vi "Curtin1_Search.vi"(9 "Old Files":T3[](array[typedef])) -> (1 "New Files":T3[](array[typedef]), 3 "Ok?":bool)   [LabVIEW 2022 SP3]
uses:
  Curtin1_Label.ctl
  <vilib>/Utility/miscctls.llb/LVSelectionTypeDef.ctl
panel:
  in  "Listing Order":T1(ring)
  in  "Tags":T2={"Pattern (eg. H,V)"="H,V", "File type"={"AvR"=TRUE, "AvC"=FALSE, "trf"=FALSE, "wav"=FALSE, "All"=FALSE}, "keywords 1"="", "keywords 2"="", "keywords 3"=""}
  out "# Files":i32
  out "AllFiles":path[](array[path])
  in  "Options":i32[](listbox)
  out "Files":path[](array[path])
  in  "Dialog":bool
  out "Subfolder":string
  in  "Search":bool
  out "Folder":cluster{"Folder Path":path, "tags":string[]}[](array[cluster])
  out "List":string
  in  "Cancel Button":bool
  in  "OK Button":bool
  # "Or"
  # "Or"
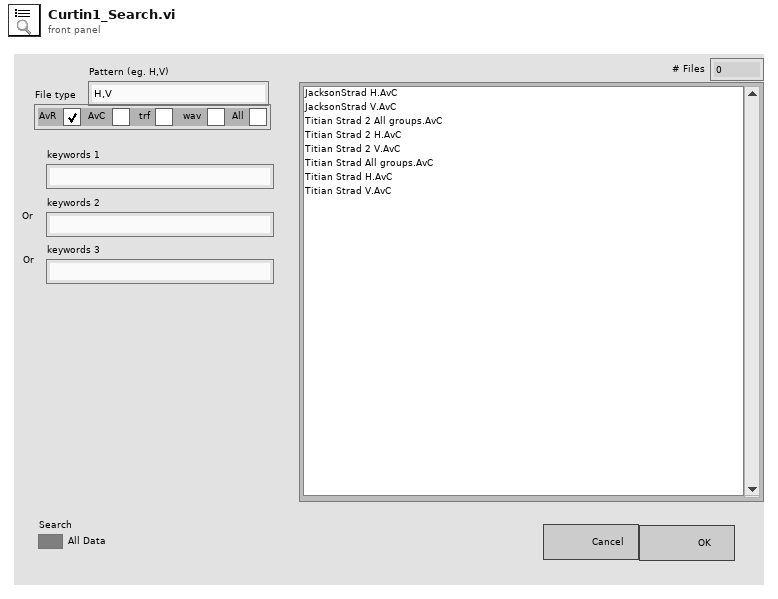
[diagram p1: front panel]
types:
  T1 = enum16{"Alphabetical", "Chronological", "Hit Strength (min to max)", "Hit Strength (max to min)"}
  T2 = cluster{"Pattern (eg. H,V)":string, "File type":cluster{"AvR":bool, "AvC":bool, "trf":bool, "wav":bool, "All":bool}, "keywords 1":string, "keywords 2":string, "keywords 3":string}
  T3 = typedef "Curtin1_Label.ctl" = cluster{"Show?":bool, "Name":string, "Color":u32, "Path":path, "Show Notes":bool}
  T4 = typedef "LVSelectionTypeDef.ctl" = cluster{"Selection Start":u32, "Selection End":u32}
  T5 = cluster{"Pattern (eg. H,V)":string, "File type":cluster{"AvR":bool, "AvC":bool, "trf":bool, "wfm":bool, "All":bool}, "keywords 1":string, "keywords 2":string, "keywords 3":string}
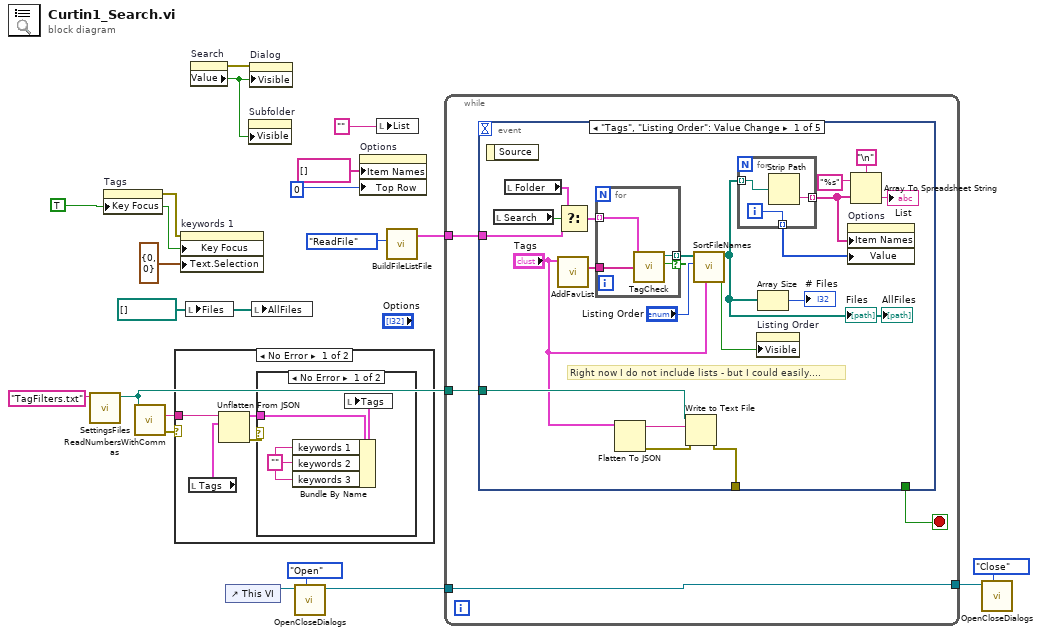
[diagram p0: block diagram]
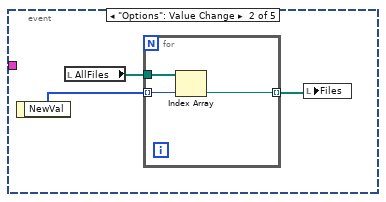
[diagram p4: hidden frame]
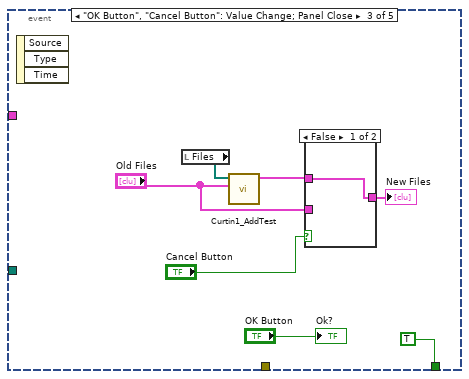
[diagram p5: hidden frame]
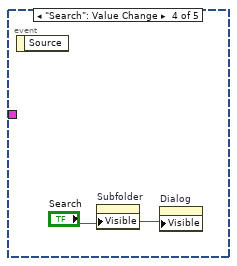
[diagram p7: hidden frame]
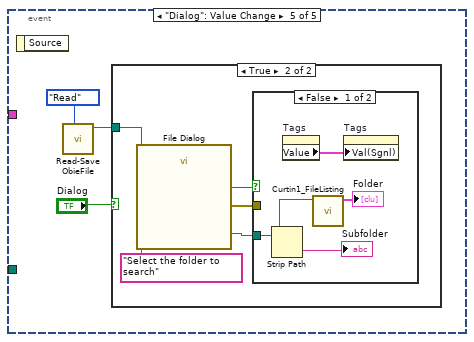
[diagram p8: hidden frame]
diagram:
  w3 = path[] [] ("Files")
  w12 = TRUE ("Visible")
  n1 = call "SettingsFiles.vi"("settings file name"="TagFilters.txt" ("name or relative path")) -> ("file path"=w1:path)  [unwired: 9 in, 1 out]
  n2 = property on="Tags" class="Clust (strict)"("Key Focus"=w12) -> (error out=w11:errorcluster)  [unwired: 2 in, 1 out]
  n3 = call "ReadNumbersWithCommas.vi"("file (use dialog)"=w1) -> ("error out"=w9:errorcluster, "text"=w10:string)  [unwired: 7 in, 2 out]
  n4 = case shown="No Error" w9 {
    tunnel: w10 -> [w23 _]
    frame No Error {
      n5 = local read "Tags"() -> (w24:T2)
      n6 = Unflatten From JSON(JSON string=w23, type and defaults=w24) -> (value=w21:T2, error out=w22:errorcluster)  [unwired: 5 in]
      n7 = case shown="No Error" w22 {
        tunnel: w21 -> [w27 _]
        frame No Error {
          w26 = "" ("Tags 1")
          n8 = Bundle By Name(cluster=w27, "keywords 1"=w26, "keywords 2"=w26, "keywords 3"=w26) -> (w25:T2)
          n9 = local write "Tags"(w25) -> ()
        }
        frame Error {
        }
      }
    }
    frame Error {
    }
  }
  n10 = property on="keywords 1" class="Str"(error in=w11, "Key Focus"=w12, "Text.Selection"=T4 {"Selection Start"=0, "Selection End"=0}) -> ()  [unwired: 1 in, 2 out]
  n11 = local write "Files"(w3) -> ()
  n12 = property on="Search" class="Bool (strict)"() -> (error out=w16:errorcluster, "Value"=w15:bool)  [unwired: 2 in, 1 out]
  n13 = control-ref of="This VI"() -> (w7:refnum<vi>)
  n14 = property on="Subfolder" class="Str"("Visible"=w15) -> ()  [unwired: 2 in, 2 out]
  n15 = property on="Dialog" class="Bool"(error in=w16, "Visible"=w15) -> ()  [unwired: 1 in, 2 out]
  n16 = local write "AllFiles"(w3) -> ()
  n17 = call "OpenCloseDialogs.vi"("Task"=enum16{"Open", "Close"}."Open", "VI in"=w7) -> ("VI out"=w4:refnum<vi>)  [unwired: 8 in, 1 out]
  n18 = property on="Options" class="LstBox (strict)"("Item Names"=string[] [], "Top Row"=0) -> ()  [unwired: 2 in, 2 out]
  n19 = local write "List"("" ("List")) -> ()
  n20 = call "BuildFileListFile.vi"("Task"=enum16{"BuildFile", "ReadFile"}."ReadFile") -> ("Instruments"=w17:cluster{"Folder Path":path, "tags":string[]}[])  [unwired: 9 in, 1 out]
  n21 = while {
    tunnel: w17 -> [w30]
    tunnel: w1 -> [w29]
    tunnel: [w28] -> w5
    tunnel: w4 -> [w28]
    stop <- w31 stop-if-true
    n22 = event shown="[0] \"Tags\", \"Listing Order\": Value Change" {
      selector: _ -> [_ _ _ _ _]
      dyn-events: _ -> [_ _ _ _ _]
      timeout: _ -> [_ _ _ _ _]
      tunnel: [_ _ TRUE _ _] -> w31
      tunnel: w30 -> [w39 _ _ _ _]
      tunnel: w29 -> [w45 _ _ _ _]
      tunnel: [w43 _ _ _ _] -> _
      event "Tags", "Listing Order": Value Change {
        # "Right now I do not include lists - but I could easily...."
        n23 = event-data() -> ()  [unwired: 1 in, 1 out]
        n24 = local read "Search"() -> (w40:bool)
        n25 = local read "Folder"() -> (w38:cluster{"Folder Path":path, "tags":string[]}[])
        n26 = call "AddFavList.vi"("Tags"="Tags") -> ("Tags"=w50:string[])  [unwired: 8 in, 2 out]
        n27 = Select(t=w38, s=w40, f=w39) -> (s? t:f=w37:cluster{"Folder Path":path, "tags":string[]}[])
        n28 = for {
          tunnel: w50 -> [w56]
          tunnel: [w58] -> w36 mode=indexing if=w57
          tunnel: w37 -> [w55] mode=indexing
          n29 = call "TagCheck.vi"("Tags"=w56, 11:w55) -> ("Good?"=w57:bool, "Path out"=w58:path)  [unwired: 8 in]
        }
        n30 = Flatten To JSON(anything="Tags") -> (JSON string=w46:string, 11:w44:errorcluster)  [unwired: 2 in]
        n31 = Write to Text File(file (use dialog)=w45, text=w46, error in=w44) -> (error out=w43:errorcluster)  [unwired: 1 in, 2 out]
        n32 = call "SortFileNames.vi"("Tags"="Tags", "Listing Order"="Listing Order", "Files in"=w36) -> ("wfm only?"=w32:bool, "Files out"=w35:path[])  [unwired: 7 in]
        "Files" <- w35
        "AllFiles" <- w35
        n33 = for {
          tunnel: w35 -> [w54] mode=indexing
          tunnel: [w53] -> w42 mode=indexing
          tunnel: [w52] -> w41 mode=indexing
          i -> [w52]
          n34 = Strip Path(path=w54) -> (name=w53:string)  [unwired: 1 out]
        }
        n35 = property on="Listing Order" class="Enum (strict)"("Visible"=w32) -> ()  [unwired: 2 in, 2 out]
        n36 = Array Size(array=w35) -> (size(s)=→"# Files":i32)
        n37 = property on="Options" class="LstBox (strict)"("Item Names"=w42, "Value"=w41) -> ()  [unwired: 2 in, 2 out]
        n38 = Array To Spreadsheet String(delimiter (Tab)="\n", array=w42, 3:"%s" ("format string")) -> (spreadsheet string=→"List":string)
      }
      event "Options": Value Change {
        n39 = event-data() -> ("NewVal"=w60:i32[])  [unwired: 1 in]
        n40 = local read "AllFiles"() -> (w61:path[])
        n41 = for {
          tunnel: w61 -> [w64]
          tunnel: w60 -> [w63] mode=indexing
          tunnel: [w62] -> w59 mode=indexing
          n42 = Index Array(array=w64, index=w63) -> (element=w62:path)
        }
        n43 = local write "Files"(w59) -> ()
      }
      event "OK Button", "Cancel Button": Value Change; Panel Close {
        n44 = event-data() -> ()  [unwired: 1 in, 3 out]
        n45 = local read "Files"() -> (w71:path[])
        n46 = call "Curtin1_AddTest.vi"("Old Files"="Old Files", "Selected Paths"=w71) -> ("New Files"=w68:T3[])  [unwired: 9 in]
        n47 = case shown="False" "Cancel Button" {
          tunnel: "Old Files" -> [_ w73]
          tunnel: w68 -> [w72 _]
          tunnel: [w72 w73] -> w67
          frame False {
          }
          frame True {
          }
        }
        "New Files" <- w67
        "Ok?" <- "OK Button"
      }
      event "Search": Value Change {
        n48 = event-data() -> ()  [unwired: 1 in, 1 out]
        n49 = property on="Subfolder" class="Str"("Visible"="Search") -> ()  [unwired: 2 in, 2 out]
        n50 = property on="Dialog" class="Bool"("Visible"="Search") -> ()  [unwired: 2 in, 2 out]
      }
      event "Dialog": Value Change {
        n51 = event-data() -> ()  [unwired: 1 in, 1 out]
        n52 = call "Read-Save ObieFile.vi"("Task"=enum16{"Save", "Read"}."Read") -> ("DataPath Out"=w75:path)  [unwired: 8 in, 2 out]
        n53 = case shown="True" "Dialog" {
          tunnel: w75 -> [_ w79]
          frame False {
          }
          frame True {
            n54 = call "File Dialog"("start path"=w79, "prompt"="Select the folder to search" ("List")) -> ("selected path"=w82:path, "cancelled"=w81:bool, "error out"=w80:errorcluster)  [unwired: 10 in, 1 out]
            n55 = case shown="False" w81 {
              tunnel: w82 -> [w85 _]
              tunnel: w80 -> [_ _]
              frame False {
                n56 = Strip Path(path=w85) -> (name=→"Subfolder":string)  [unwired: 1 out]
                n57 = property on="Tags" class="Clust (strict)"() -> ("Value"=w83:T5)  [unwired: 2 in, 2 out]
                n58 = call "Curtin1_FileListing.vi"("Folder Path"=w85) -> ("Array"=→"Folder":cluster{"Folder Path":path, "tags":string[]}[])  [unwired: 10 in]
                n59 = property on="Tags" class="Clust (strict)"("Val(Sgnl)"=w83) -> ()  [unwired: 2 in, 2 out]
              }
              frame True {
              }
            }
          }
        }
      }
    }
  }
  n60 = call "OpenCloseDialogs.vi"("Task"=enum16{"Open", "Close"}."Close", "VI in"=w5) -> ()  [unwired: 8 in, 2 out]
